vi "UI_AutoRefresh_Do(DVR).vi"(8 "error in (no error)":errorcluster, 9 "AR Mode (ind only)":T1=enum."Indicators only", 10 "Data DVR":refnum<data-value>, 11 "UI_Actor in":refnum<class "UI_Actor.lvclass">) -> (0 "error out":errorcluster, 3 "UI_Actor out":refnum<class "UI_Actor.lvclass">)   [LabVIEW 2015]
uses:
  UI_Actor.lvclass
  ctl_AR_Mode.ctl
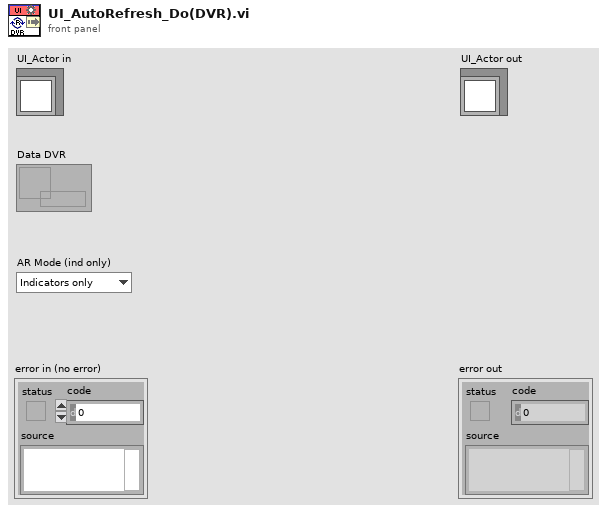
[diagram p1: front panel]
types:
  T1 = typedef "UI_Actor.lvlib/UI_Actor.lvclass/ctl_AR_Mode.ctl" = enum16{"Controls only", "Indicators only", "All"}
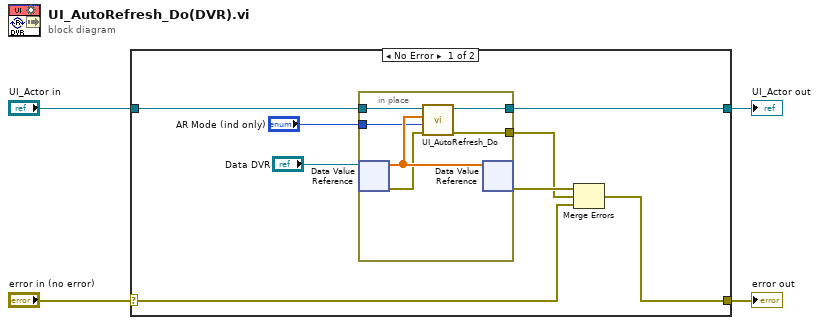
[diagram p0: block diagram]
diagram:
  n1 = case shown="No Error" "error in (no error)" {
    selector: "error in (no error)" -> [w7 w20]
    tunnel: [w6 w20] -> w3
    tunnel: [w10 w19] -> w1
    tunnel: "UI_Actor in" -> [w11 w19]
    frame No Error {
      n2 = in-place {
        in-place-border: w11 -> [w18]
        in-place-border: [w17] -> w10
        in-place-border: [w14] -> w8
        in-place-border: "AR Mode (ind only)" -> [w13]
        n3 = in-place-dvr #1("Data DVR") -> (w16:dbl[], w15:errorcluster)
        n4 = call-dynamic "UI_AutoRefresh_Do.vi"("error in (no error)"=w15, "AR Mode (ind only)"=w13, "Data"=w16, "UI_Actor in"=w18) -> ("error out"=w14:errorcluster, "UI_Actor out"=w17:refnum<class "UI_Actor.lvclass">)  [unwired: 6 in]
        n5 = in-place-dvr #1(w16) -> (w9:errorcluster)  [unwired: 1 out]
      }
      n6 = Merge Errors(w9, w8, w7) -> (w6:errorcluster)
    }
    frame Error {
    }
  }
  "error out" <- w3
  "UI_Actor out" <- w1
